vi "Query All Hardware FPGA.vi"(0 "VISA resource name":refnum<visa-resource-name>, 5 "Query Type All (0: Hardware)":u16(ring) items=["Hardware", "FPGA"], 11 "error in (no error)":errorcluster) -> (4 "VISA resource name out":refnum<visa-resource-name>, 8 "Revision Information":cluster{"Hardware":string, "Revision":i32}[](array[cluster]), 15 "error out":errorcluster)   [LabVIEW 2020, in "Anritsu Signal Analyzer Series.lvlib"]
doc: "Queries the revision number of all the hardware or all FPGA."
uses:
  Anritsu Signal Analyzer Series.lvlib
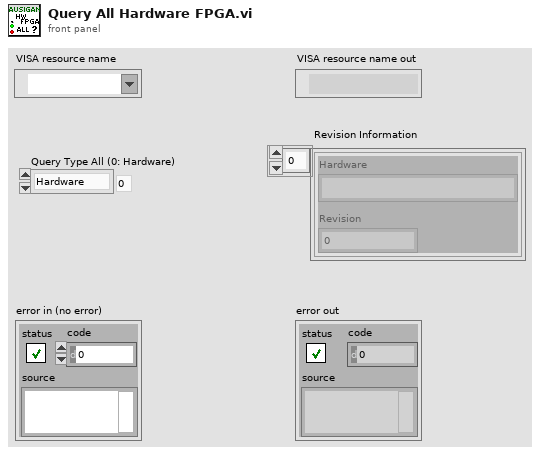
[diagram p1: front panel]
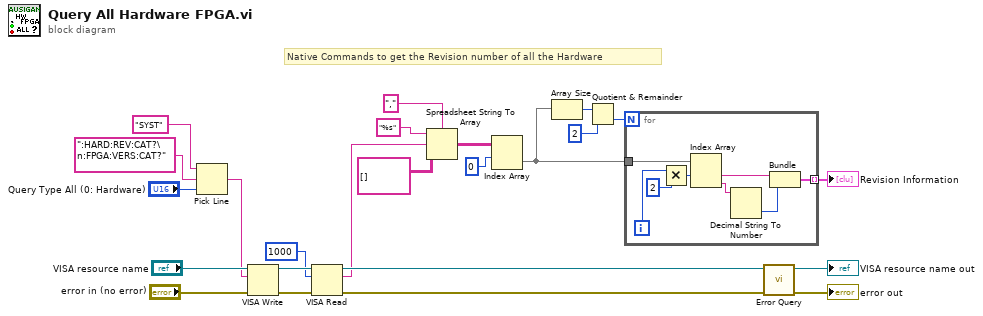
[diagram p0: block diagram]
diagram:
  # "Native Commands to get the Revision number of all the Hardware"
  n1 = Pick Line(string ("")="SYST", multi-line string=":HARD:REV:CAT?\n:FPGA:VERS:CAT?", line index="Query Type All (0: Hardware)") -> (output string=w2:string)
  n2 = VISA Write(VISA resource name="VISA resource name", write buffer=w2, error in (no error)="error in (no error)") -> (VISA resource name out=w22:refnum<visa-resource-name>, error out=w21:errorcluster)  [unwired: 1 out]
  n3 = VISA Read(VISA resource name=w22, byte count=u32 1000 ("byte count (0)"), error in (no error)=w21) -> (VISA resource name out=w16:refnum<visa-resource-name>, read buffer=w15:string, error out=w17:errorcluster)  [unwired: 1 out]
  n4 = Spreadsheet String To Array(delimiter (Tab)=",", format string="%s", spreadsheet string=w15, array type (2D Dbl)=string[][] []) -> (array=w11:string[][])
  n5 = Index Array(array=w11, index (row)=0) -> (element=w8:string[])  [unwired: 1 in]
  n6 = Array Size(array=w8) -> (size(s)=w7:i32)
  n7 = Quotient & Remainder(x=w7, y=2) -> (floor(x/y)=w5:i32)  [unwired: 1 out]
  n8 = for {
    N: w5 -> [_]
    tunnel: w8 -> [w32]
    tunnel: [w27] -> w9 mode=indexing
    i -> [w31]
    n9 = Multiply(x=w31, y=2) -> (x*y=w29:i32)
    n10 = Index Array(array=w32, index #1=w29) -> (element #1=w28:string, element #2=w26:string)  [unwired: 1 in]
    n11 = Decimal String To Number(string=w26) -> (number=w25:i32)  [unwired: 2 in, 1 out]
    n12 = Bundle(w28, w25) -> (w27:cluster{string, i32})  [unwired: 1 in]
  }
  "Revision Information" <- w9
  n13 = call "Error Query.vi"("error in (no error)"=w17, "VISA resource name"=w16) -> ("error out"=→"error out":errorcluster, "VISA resource name out"=→"VISA resource name out":refnum<visa-resource-name>)  [unwired: 6 in, 2 out]
